vi "Topo & GridSpectr_DriftCorrection_v8.vi"(6 "Internal use":string, 7 "Grid param":T2 {"height (m)" format="%#_6p"; "width (m)" format="%#_6p"; "center Y (m)" format="%#_6p"; "center X (m)" format="%#_6p"}, 8 "Error in (no error)":errorcluster, 9 "Points Y/Index Y":i32, 10 "Points X/Index X":i32, 11 "Method":enum16{"init", "run", "end"}(ring)=enum."end") -> (0 "Error out":errorcluster)   [LabVIEW 2014]
doc: "Example of a measurement VI to be used in the \"Experiments on a Grid\" tool as external VI.\n\nThis example measure the topography and spectroscopy data. The spectroscopy measurements are taken on a subgrid. The data are saved to a sxm and a binary file.\n\n- Nanonis Programming Interface -"
uses:
  <userlib>/Nanonis Prog Interface V5/Nanonis Prog Interface.lvlib
  <userlib>/Nanonis Prog Interface V5/Scan/Grid/GridPatternGet.vi
panel:
  out "Progress":u8(slide) scale=0.0..100.0 scale format="%#.1g"
  out "total Points":i32
  in  "preSTS delay [ms]":u32=3
  in  "STS Bias":dbl=0.005 format="%#_6p"
  in  "Move Bias":dbl=-0.01 format="%#_6p"
  in  "Move Current":dbl=1.5e-11 format="%#_6p"
  in  "Imaging Bias":dbl=-0.01 format="%#_6p"
  in  "max applied Drift Correction":i32=20 min=1 max=100 step=1 format="%.0p"
  in  "Correlate":u16(ring) items=["first Frame", "successive Frames"]
  out "Topo Images taken":i32=14
  in  "Increment":i32=40
  in  "Threshold":i32=2 min=1 step=1
  in  "tip Speed (m/s)":sgl=1e-08 format="%.2p"
  in  "Drift Correction 2":T1
  out "X drift":i32
  out "Y drift":i32
  out "Last Drift detected":i32=40
  in  "MaxImagesBack":i32=40
  in  "Channel index (0-23)":u8=14
  in  "File name":string="single_mol_shortSTS"
  in  "STS Current":dbl=1.15e-09 format="%#_6p"
  in  "Imaging Current":dbl=1.5e-11 format="%#_6p"
  in  "zdrift \nDuration (s)":dbl
  in  "Correct z drift":bool
  out "Status":string="finishing"
  in  "Drift correction Pixels":i32=256 caption="Topo Pixels"
  out "Y Offset":dbl format="%#_6p"
  out "X Offset":dbl format="%#_6p"
  out "Points taken":dbl=14.0
  in  "Drift Correction every":i32=40
  in  "Y subgrid spacing":u16=1
  in  "X subgrid spacing":u16=1
  # "GRID points"
  # "Increase this if no Drift was detected for \na certain number of images"
  # "images back"
  # "% of image size"
  # "RUN smart tilt before starting the GRID"
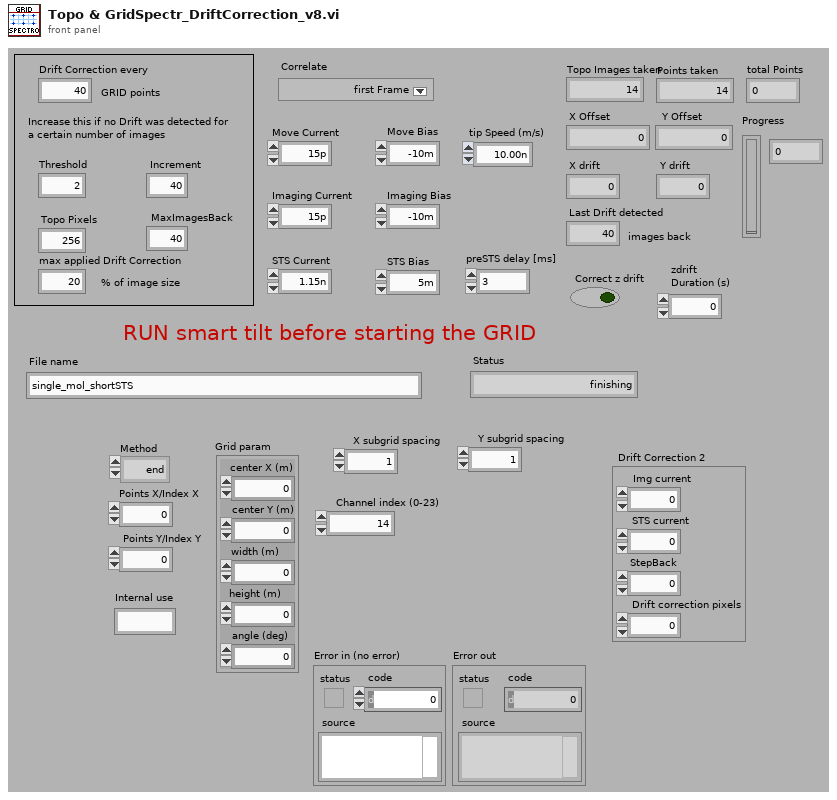
[diagram p1: front panel]
types:
  T1 = cluster{"Img current":dbl, "STS current":dbl, "StepBack":dbl, "Drift correction pixels":dbl}
  T2 = cluster{"center X (m)":sgl, "center Y (m)":sgl, "width (m)":sgl, "height (m)":sgl, "angle (deg)":sgl}
  T3 = cluster{"center X":sgl, "center Y":sgl, "angle":sgl, "width":sgl, "height":sgl, "# pixels":i32, "# lines":i32}
  T4 = cluster{"Name":string, "Calibration":sgl, "Offset":sgl, "Channel index":i32}[]
  T5 = cluster{"up/down":bool, "time/line":sgl, "start time":timestamp, "end time":timestamp}
  T6 = cluster{"Z averaging time (s)":sgl, "Z offset (m)":sgl, "Initial settling time (s)":sgl}
  T7 = cluster{"Max. slew rate (V/s)":sgl, "Settling time (s)":sgl, "Integration time (s)":sgl}
  T8 = cluster{"End settling time (s)":sgl, "Z control time (s)":sgl}
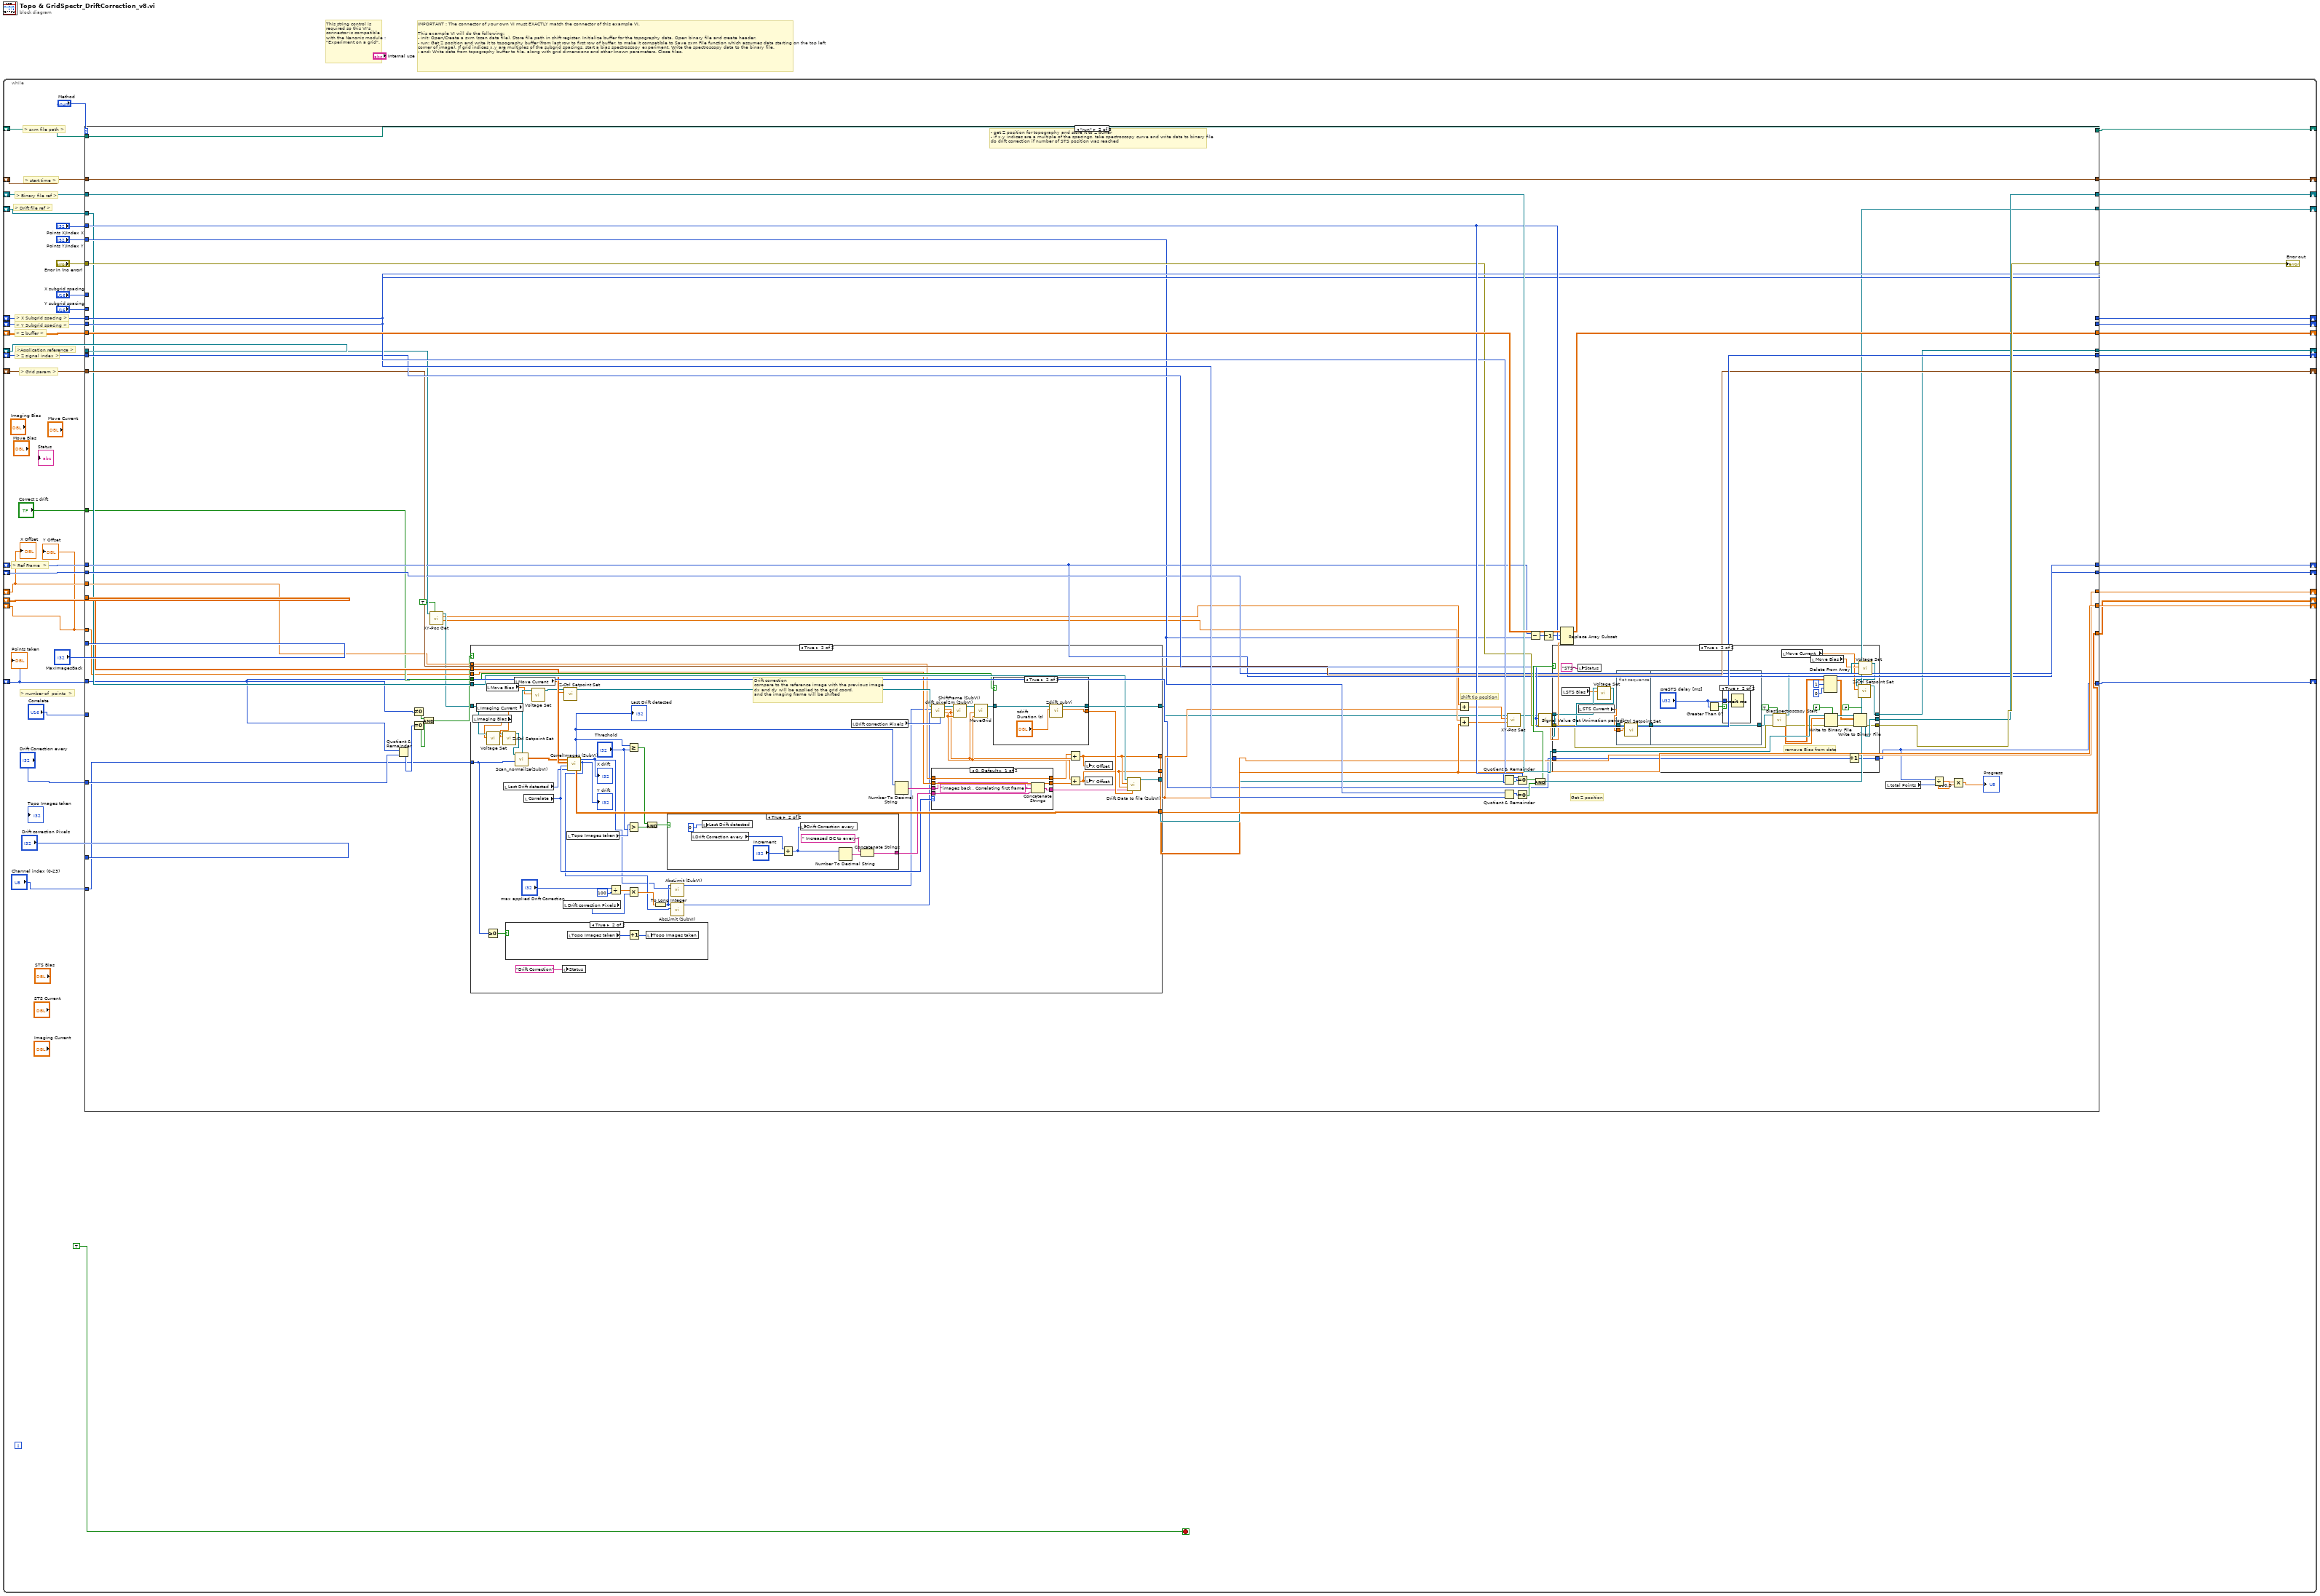
[diagram p0: block diagram]
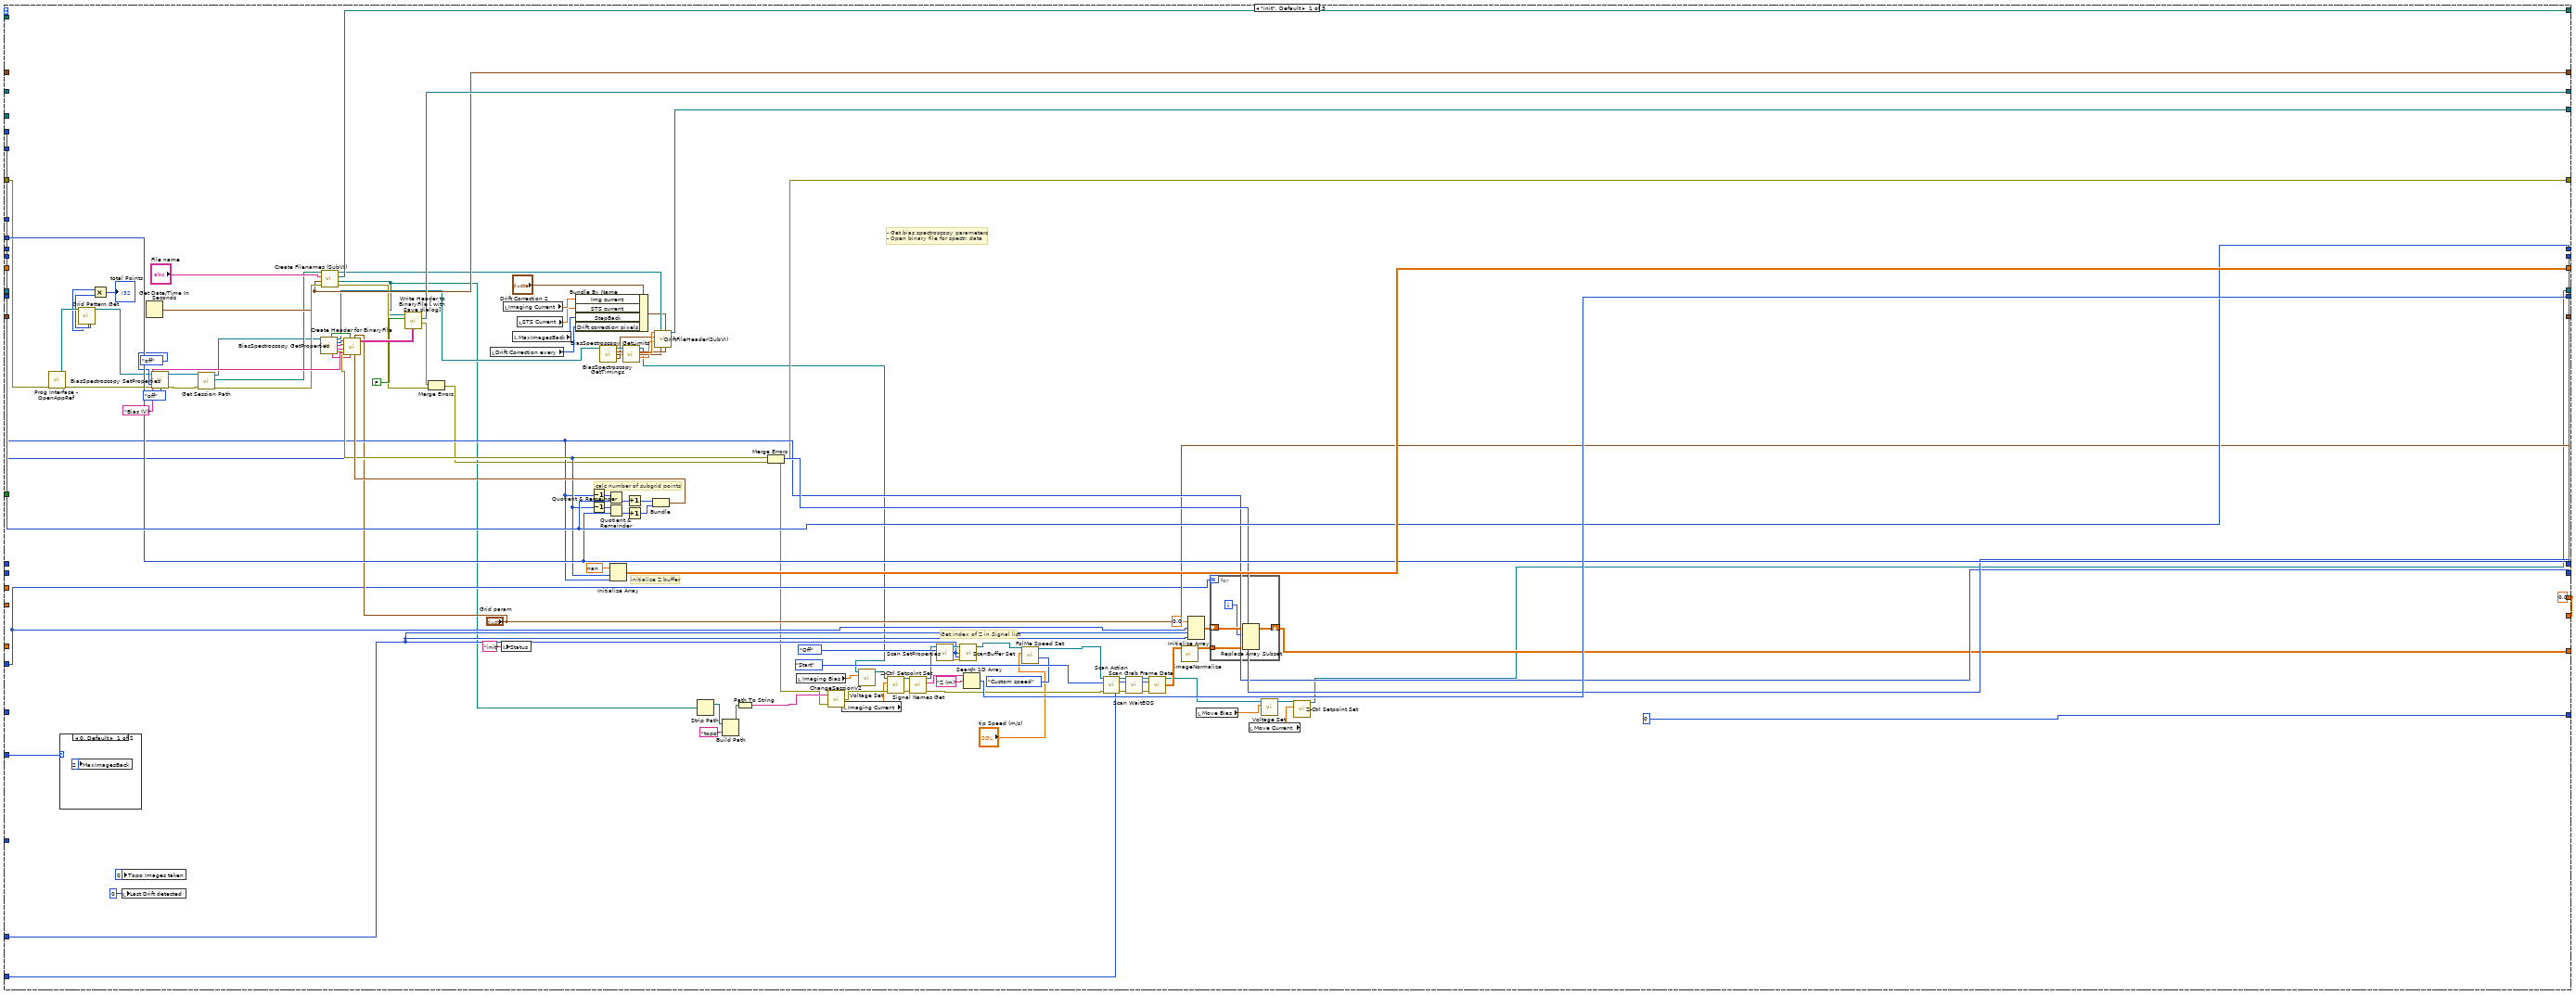
[diagram p2: hidden frame]
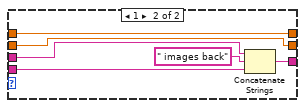
[diagram p5: hidden frame]
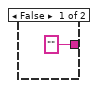
[diagram p7: hidden frame]
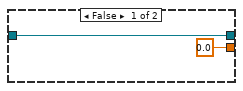
[diagram p8: hidden frame]
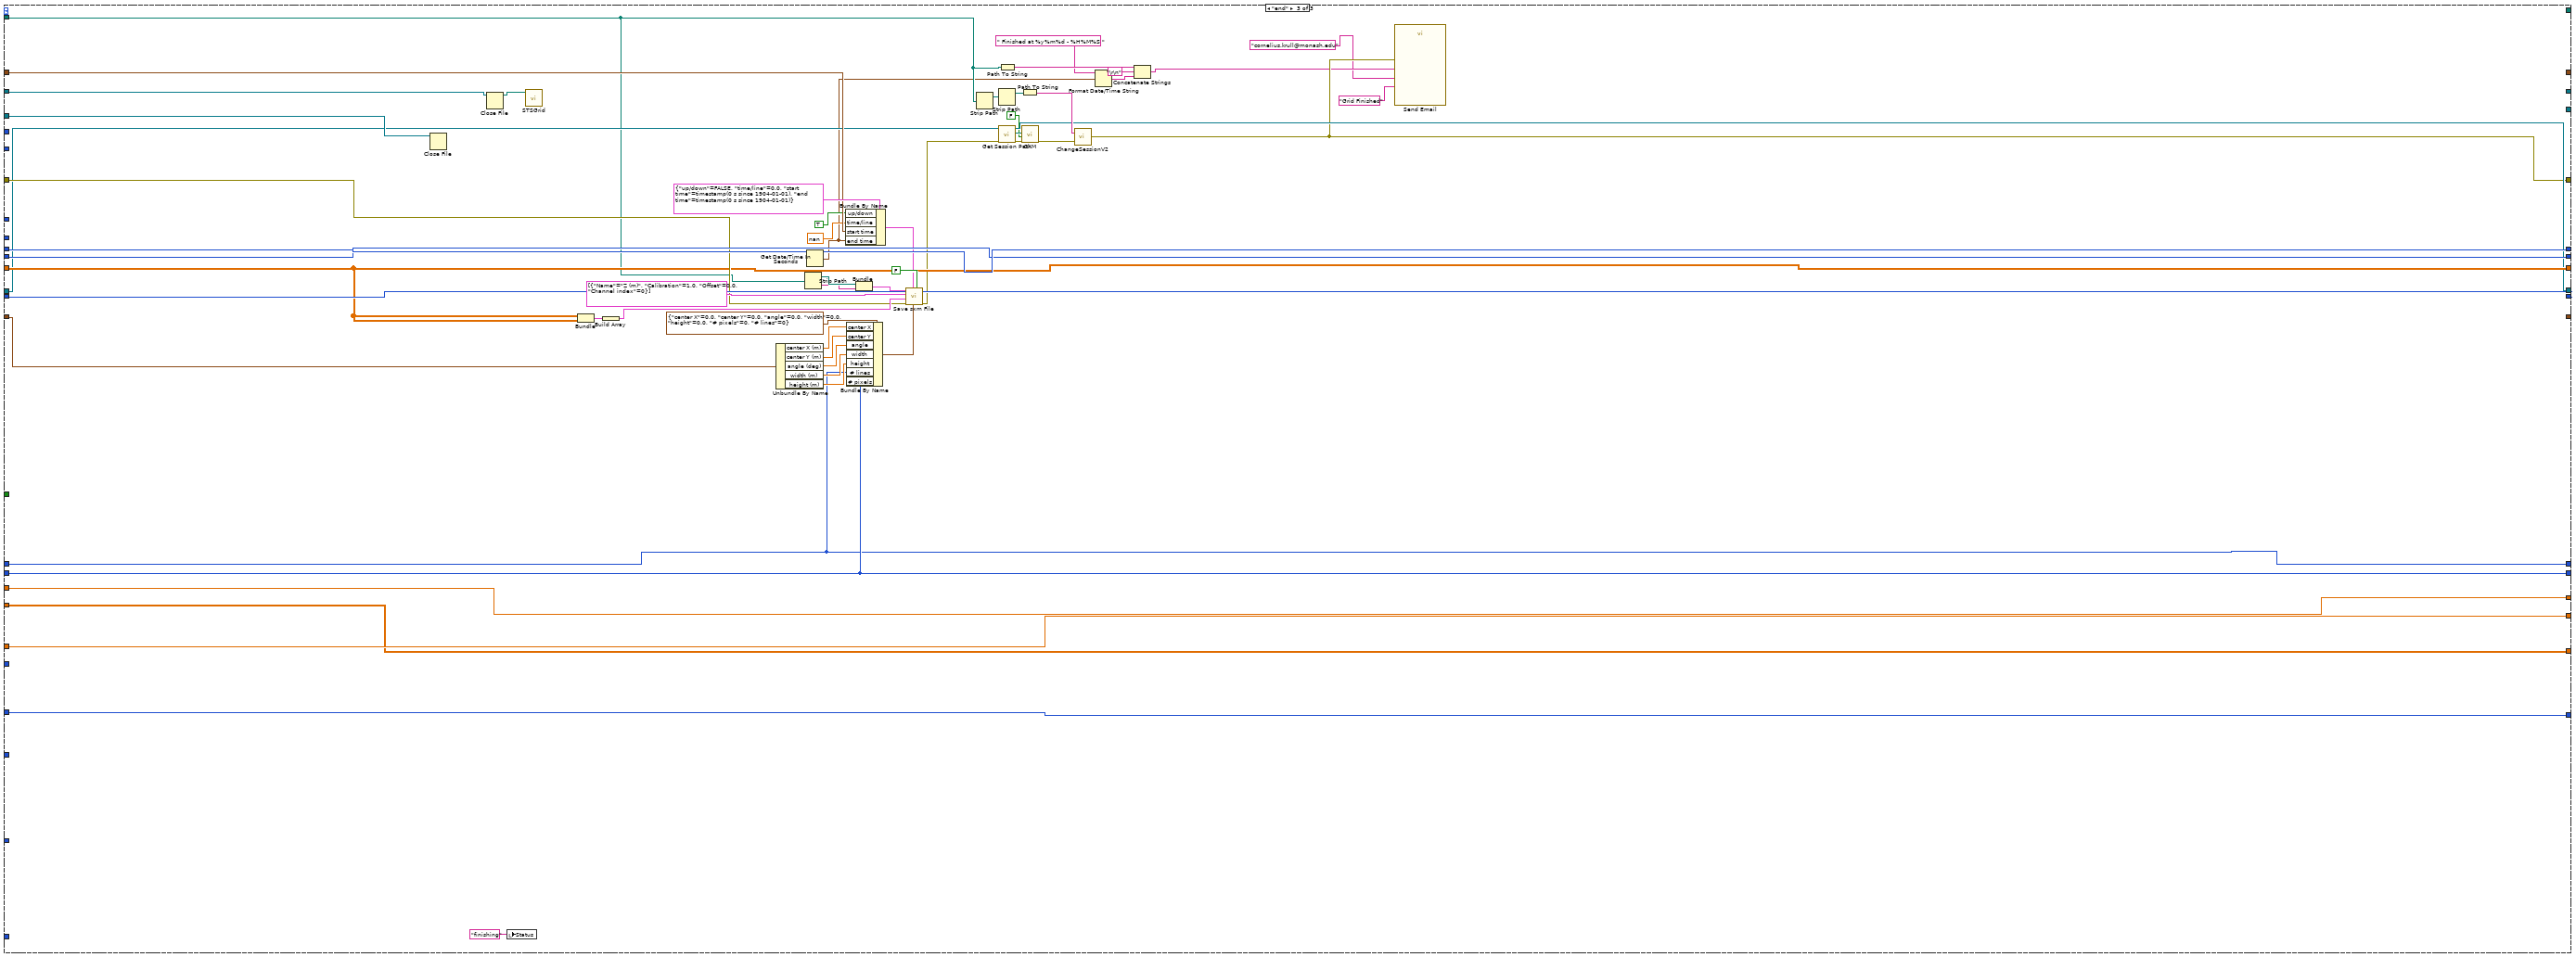
[diagram p11: hidden frame]
diagram:
  # "This string control is required so this VI's connector is compatible with the Nanonis module : \"Experiment on a grid\"."
  # "IMPORTANT : The connector of your own VI must EXACTLY match the connector of this example VI.\n\nThis example VI will do the following:\n- init: Open/Create a sxm (scan data file). Store file path in shift register. Initialize buffer for the topography data. Open binary file and create header.\n- run: Get Z position and write it to topography buffer (from last row to first row of buffer, to make it compatible to Save sxm File function which assumes data starting on the top left corner of image). If grid indices x,y are multiples of the subgrid spacings, start a bias spectroscopy experiment. Write the spectroscopy data to the binary file.\n- end: Write data from topography buffer to file, along with grid dimensions and other known parameters. Close files."
  n1 = while {
    shift-right: [w21] -> _
    shift-left: _ -> [w44]
    shift-right: [w39] -> _
    shift-left: _ -> [w38]
    shift-right: [w36] -> _
    shift-left: _ -> [w37]
    shift-right: [w35] -> _
    shift-left: _ -> [w34]
    shift-right: [w28] -> _
    shift-left: _ -> [w30]
    shift-right: [w29] -> _
    shift-left: _ -> [w31]
    shift-right: [w27] -> _
    shift-left: _ -> [w26]
    shift-right: [w25] -> _
    shift-left: _ -> [w24]
    shift-right: [w23] -> _
    shift-left: _ -> [w22]
    shift-right: [w20] -> _
    shift-left: _ -> [w19]
    shift-right: [w18] -> _
    shift-left: _ -> [w17]
    shift-right: [w16] -> _
    shift-left: _ -> [w9]
    shift-right: [w15] -> _
    shift-left: _ -> [w8]
    shift-right: [w14] -> _
    shift-left: _ -> [w11]
    shift-right: [w13] -> _
    shift-left: _ -> [w10]
    shift-right: [w6] -> _
    shift-left: _ -> [w5]
    stop <- TRUE stop-if-true
    # "> Drift file ref >"
    # "> number of  points  >"
    # "> Ref Frame  >"
    # "> Grid param >"
    # "> start time >"
    # ">Application reference >"
    # "> Y Subgrid spacing >"
    # "> X Subgrid spacing >"
    # "> Z signal index >"
    # "> Binary file ref >"
    # "> Z buffer >"
    # "> sxm file path >"
    n2 = case shown="\"run\"" "Method" {
      tunnel: [w109 w216 _] -> w21
      tunnel: w44 -> [_ w216 w352]
      tunnel: "Error in (no error)" -> [w111 w202 w384]
      tunnel: [w72 w215 w353] -> w42
      tunnel: "Points X/Index X" -> [w130 w210 _]
      tunnel: "Points Y/Index Y" -> [w131 w194 _]
      tunnel: [w154 w213 w373] -> w39
      tunnel: w38 -> [_ w214 w373]
      tunnel: w37 -> [_ w212 w366]
      tunnel: [w146 w211 _] -> w36
      tunnel: [w144 w200 w398] -> w35
      tunnel: w34 -> [_ w200 w398]
      tunnel: "X subgrid spacing" -> [w143 _ _]
      tunnel: "Y subgrid spacing" -> [w142 _ _]
      tunnel: w31 -> [_ w204 w397]
      tunnel: w30 -> [_ w203 w396]
      tunnel: [w143 w204 w397] -> w29
      tunnel: [w142 w203 w396] -> w28
      tunnel: [w60 w187 w358] -> w27
      tunnel: w26 -> [_ w170 w359]
      tunnel: ["Grid param" w197 _] -> w25
      tunnel: w24 -> [_ w197 w383]
      tunnel: [w108 w198 _] -> w23
      tunnel: w22 -> [_ w198 w391]
      tunnel: [w131 w195 w374] -> w20
      tunnel: w19 -> [_ w195 w374]
      tunnel: [w130 w196 w375] -> w18
      tunnel: w17 -> [_ w196 w375]
      tunnel: [w121 w177 w372] -> w16
      tunnel: [w121 w182 w370] -> w15
      tunnel: [w103 w176 w367] -> w14
      tunnel: [0 w164 w371] -> w13
      tunnel: w10 -> [_ w173 w371]
      tunnel: "Drift Correction every" -> [_ w190 _]
      tunnel: w11 -> [_ w181 w367]
      tunnel: w9 -> [_ w188 w372]
      tunnel: w8 -> [_ w174 w370]
      tunnel: "Drift correction Pixels" -> [w102 _ _]
      tunnel: [w98 w179 _] -> w6
      tunnel: w5 -> [_ w180 w368]
      tunnel: "Correct z drift" -> [_ w178 _]
      tunnel: "Channel index (0-23)" -> [w106 w175 _]
      tunnel: "MaxImagesBack" -> [w101 _ _]
      tunnel: "Correlate" -> [w63 _ _]
      frame "init", Default {
        w121 = 0.0
        # "- Get bias spectroscopy parameters\n- Open binary file for spectr. data"
        # "initialize Z buffer"
        # "calc number of subgrid points"
        # "Get index of Z in Signal list"
        n3 = call <userlib>:"Prog Interface - OpenAppRef.vi"("Error in (no error)"=w111) -> ("Error out"=w70:errorcluster, "Application reference"=w51:refnum<vi>)  [unwired: 5 in]
        n4 = case shown="0, Default" w63 {
          frame 0, Default {
            n5 = local write "MaxImagesBack"(2 ("StepsBack")) -> ()
          }
          frame 1 {
          }
        }
        n6 = call-poly <userlib>:"Grid Pattern Get.vi"("Application ref in"=w51) -> ("Points Y"=w48:i32, "Points X"=w49:i32, "Application ref out"=w50:refnum<vi>)  [unwired: 10 in, 6 out]
        n7 = Multiply(x=w48, y=w49) -> (x*y=→"total Points":i32)
        n8 = local write "Topo Images taken"(0 ("Images taken")) -> ()
        n9 = local write "Last Drift detected"(0 ("Last Drift detected")) -> ()
        n10 = Get Date/Time In Seconds() -> (seconds since 1Jan1904=w108:timestamp)
        n11 = call <userlib>:"BiasSpectroscopy SetProperties.vi"("Application ref in"=w50, "Autosave (no change)"=enum16{"no change", "on", "off"}."off", "Error in (no error)"=w70, "Save dialog"=enum16{"no change", "on", "off"}."off") -> ("Application ref out"=w66:refnum<vi>, "Error out"=w65:errorcluster)  [unwired: 10 in]
        n12 = call <userlib>:"Get Session Path.vi"("error in (no error)"=w65, "Application ref in"=w66) -> ("error out"=w110:errorcluster, "Session path"=w78:path, "Application ref out"=w67:refnum<vi>)  [unwired: 7 in]
        n13 = call <userlib>:"BiasSpectroscopy GetProperties.vi"("Application ref in"=w67) -> ("Backward sweep"=w150:bool, "Application ref out"=w82:refnum<vi>, "Number of points"=w133:i32, "Channels"=w132:string[], "Parameters"=w148:string[], "Fixed parameters"=w135:string[], "Error out"=w147:errorcluster)  [unwired: 6 in, 2 out]
        n14 = call "Create Filenames (SubVI).vi"("error in (no error)"=w110, "seconds since 1Jan1904"=w108, "File name"="File name", "Session path"=w78) -> ("error out"=w83:errorcluster, "binFilePath"=w74:path, "topoFilePath"=w109:path, "Drift File out"=w99:refnum<file>)  [unwired: 4 in]
        n15 = local read "Drift Correction every"() -> (w93:i32)
        n16 = local write "Status"("init" ("Status")) -> ()
        n17 = local read "Imaging Current"() -> (w95:dbl)
        n18 = local read "MaxImagesBack"() -> (w92:i32)
        n19 = local read "STS Current"() -> (w94:dbl)
        n20 = Bundle By Name(cluster="Drift Correction 2", "Img current"=w95, "STS current"=w94, "StepBack"=w92, "Drift correction pixels"=w93) -> (w96:T1)
        n21 = Decrement(x=w130) -> (x-1=w141:i32)
        n22 = Decrement(x=w131) -> (x-1=w140:i32)
        n23 = call <userlib>:"BiasSpectroscopy GetTimings.vi"("Application ref in"=w82) -> ("Application ref out"=w91:refnum<vi>, "Initialization"=w88:T6, "Sweep Timing"=w86:T7, "End of Sweep"=w87:T8)  [unwired: 10 in, 1 out]
        n24 = Quotient & Remainder(x=w141, y=w143) -> (floor(x/y)=w139:i32)  [unwired: 1 out]
        n25 = Quotient & Remainder(x=w140, y=w142) -> (floor(x/y)=w138:i32)  [unwired: 1 out]
        n26 = Initialize Array(sgl nan ("element"), w131, w130) -> (w154:sgl[][])
        n27 = call <userlib>:"BiasSpectroscopy GetLimits.vi"("Application ref in"=w91) -> ("End value (V)"=w89:sgl, "Start value (V)"=w90:sgl, "Application ref out"=w58:refnum<vi>)  [unwired: 5 in, 1 out]
        n28 = Increment(x=w139) -> (x+1=w137:i32)
        n29 = Increment(x=w138) -> (x+1=w136:i32)
        n30 = Bundle(w137, w136) -> (w149:cluster{i32, i32})  [unwired: 1 in]
        n31 = call <userlib>:"Create Header for BinaryFile.vi"("Grid points"=w149, "Grid param"="Grid param", "Fixed parameters"=w135, "Backward sweep"=w150, "Sweep signal"="Bias (V)" ("Sweep Signal"), "Parameters"=w148, "Channels"=w132, "Points per sweep"=w133) -> ("Header (fixed attributes)"=w152:string[][])  [unwired: 3 in]
        n32 = call <userlib>:"Write Header to BinaryFile [ with Save dialog].vi"("Fixed Attributes"=w152, "Show Dialog? (T)"=FALSE, "Filename"=w74) -> ("Error out"=w84:errorcluster, "File ref"=w146:refnum<file>)  [unwired: 5 in, 2 out]
        n33 = Merge Errors(w84, w83) -> (w85:errorcluster)
        n34 = call "DriftFileHeader(SubVI).vi"("Initialization"=w88, "Drift Correction"=w96, "Sweep Timing"=w86, "Byte Stream File in"=w99, "End value (V)"=w89, "End of Sweep"=w87, "Start value (V)"=w90) -> ("Byte Stream File out"=w98:refnum<file>)  [unwired: 4 in]
        n35 = Strip Path(path=w74) -> (stripped path=w77:path)  [unwired: 1 out]
        n36 = Build Path(base path=w77, name or relative path="topo") -> (appended path=w75:path)
        n37 = Path To String(path=w75) -> (string=w73:string)
        n38 = Merge Errors(w147, w85) -> (w72:errorcluster)
        n39 = local read "Imaging Bias"() -> (w54:dbl)
        n40 = call "ChangeSessionV2.vi"("error in (no error)"=w72, "Session"=w73) -> ("error out"=w71:errorcluster)
        n41 = local read "Imaging Current"() -> (w53:dbl)
        n42 = call <userlib>:"Voltage Set.vi"("Bias (V)"=w54, "Application ref in"=w58) -> ("Application ref out"=w57:refnum<vi>)  [unwired: 8 in, 1 out]
        n43 = call <userlib>:"Z-Ctrl Setpoint Set.vi"("error in (no error)"=w71, "Z Controller setpoint"=w53, "Application ref in"=w57) -> ("error out"=w112:errorcluster, "Application ref out"=w113:refnum<vi>)  [unwired: 7 in]
        n44 = call <userlib>:"Signal Names Get.vi"("error in (no error)"=w112, "Application ref in"=w113) -> ("error out"=w122:errorcluster, "Signals Names"=w134:string[], "Application ref out"=w117:refnum<vi>)  [unwired: 5 in]
        n45 = call <userlib>:"Scan SetProperties.vi"("Application ref in"=w117, "Continuous scan"=enum16{"No change", "On", "Off"}."Off") -> ("Application ref out"=w119:refnum<vi>, "Error out"=w118:errorcluster)  [unwired: 12 in]
        n46 = call <userlib>:"ScanBuffer Set.vi"("Application ref in"=w119, "Pixels"=w102, "Lines"=w102, "error in (no error)"=w118) -> ("Application ref out"=w61:refnum<vi>)  [unwired: 10 in, 1 out]
        n47 = Search 1D Array(1D array=w134, element="Z (m)") -> (index of element=w144:i32)  [unwired: 1 in]
        n48 = call <userlib>:"FolMe Speed Set.vi"("Speed Setting (Custom)"=enum32{"Scan speed", "Custom speed"}."Custom speed", "Speed (m/s)"="tip Speed (m/s)", "Application ref in"=w61) -> ("Application ref out"=w81:refnum<vi>)  [unwired: 5 in, 1 out]
        n49 = call <userlib>:"Scan Action.vi"("error in (no error)"=w122, "Scan action (Start)"=enum16{"Start", "Stop", "Pause", "Resume"}."Start", "Application ref in"=w81) -> ("error out"=w128:errorcluster, "Application ref out"=w127:refnum<vi>)  [unwired: 6 in]
        n50 = call <userlib>:"Scan WaitEOS.vi"("error in (no error)"=w128, "Application ref in"=w127) -> ("error out"=w125:errorcluster, "Application ref out"=w126:refnum<vi>)  [unwired: 5 in, 2 out]
        n51 = call <userlib>:"Scan Grab Frame Data.vi"("Application ref in"=w126, "Channel index (0-23)"=w106, "error in (no error)"=w125) -> ("Application ref out"=w52:refnum<vi>, "Scan frame data"=w114:sgl[][])  [unwired: 8 in, 3 out]
        n52 = call "imageNormalize.vi"("Data"=w114) -> ("Array"=w100:dbl[][])  [unwired: 10 in]
        n53 = Initialize Array(0.0 ("element"), w101, w102, w102) -> (w104:dbl[][][])
        n54 = local read "Move Bias"() -> (w56:dbl)
        n55 = for {
          N: w101 -> [_]
          tunnel: w100 -> [w158]
          shift-right: [w157] -> w103
          shift-left: w104 -> [w159]
          i -> [w156]
          n56 = Replace Array Subset(array=w159, new element=w158, index (dim 0)=w156) -> (w157:dbl[][][])  [unwired: 2 in]
        }
        n57 = local read "Move Current"() -> (w55:dbl)
        n58 = call <userlib>:"Voltage Set.vi"("Bias (V)"=w56, "Application ref in"=w52) -> ("Application ref out"=w59:refnum<vi>)  [unwired: 8 in, 1 out]
        n59 = call <userlib>:"Z-Ctrl Setpoint Set.vi"("Z Controller setpoint"=w55, "Application ref in"=w59) -> ("Application ref out"=w60:refnum<vi>)  [unwired: 8 in, 1 out]
      }
      frame "run" {
        # "shift tip position"
        # "Get Z position"
        # "- get Z position for topography and store it to Z buffer\n- if x,y indices are a multiple of the spacings, take spectroscopy curve and write data to binary file\ndo drift correction if number of STS position was reached"
        n60 = Quotient & Remainder(x=w173, y=w190) -> (x-y*floor(x/y)=w191:i32)  [unwired: 1 out]
        n61 = Not Equal To 0?(x=w173) -> (x != 0?=w171:bool)
        n62 = Equal To 0?(x=w191) -> (x = 0?=w189:bool)
        n63 = And(x=w171, y=w189) -> (x .and. y?=w172:bool)
        n64 = call <userlib>:"XY-Pos Get.vi"("Wait for newest data (F=False)"=TRUE, "Application ref in"=w170) -> ("Y (m)"=w166:sgl, "X (m)"=w167:sgl, "Application ref out"=w169:refnum<vi>)  [unwired: 5 in, 1 out]
        n65 = case shown="True" w172 {
          tunnel: w169 -> [w221 w229]
          tunnel: [w221 w271] -> w165
          tunnel: w181 -> [w218 w266]
          tunnel: [w220 w269] -> w177
          tunnel: [w219 w268] -> w182
          tunnel: w188 -> [w220 w245]
          tunnel: w174 -> [w219 w243]
          tunnel: [w218 w262] -> w176
          tunnel: w180 -> [w217 w274]
          tunnel: [w217 w273] -> w179
          tunnel: w178 -> [_ w270]
          tunnel: w175 -> [_ w249]
          frame False {
          }
          frame True {
            # "Drift correction \ncompare to the reference image with the previous image \ndx and dy will be applied to the grid coord, \nand the imaging frame will be shifted"
            n66 = local read "Imaging Bias"() -> (w227:dbl)
            n67 = local read "Imaging Current"() -> (w226:dbl)
            n68 = local read "Move Bias"() -> (w223:dbl)
            n69 = Greater Or Equal To 0?(x=w249) -> (x >= 0?=w248:bool)
            n70 = call <userlib>:"Voltage Set.vi"("Bias (V)"=w227, "Application ref in"=w229) -> ("Application ref out"=w228:refnum<vi>)  [unwired: 8 in, 1 out]
            n71 = call <userlib>:"Z-Ctrl Setpoint Set.vi"("Z Controller setpoint"=w226, "Application ref in"=w228) -> ("Application ref out"=w267:refnum<vi>)  [unwired: 8 in, 1 out]
            n72 = local read "Last Drift detected"() -> (w240:i32)
            n73 = case shown="True" w248 {
              frame False {
              }
              frame True {
                n74 = local read "Topo Images taken"() -> (w289:i32)
                n75 = Increment(x=w289) -> (x+1=w288:i32)
                n76 = local write "Topo Images taken"(w288) -> ()
              }
            }
            n77 = local read "Move Current"() -> (w222:dbl)
            n78 = call "Scan_normailze(SubVI).vi"("Channel index (0-23)"=w249, "Application in"=w267) -> ("Array"=w263:dbl[][], "Application out"=w224:refnum<vi>)  [unwired: 7 in, 1 out]
            n79 = local read "Correlate"() -> (w246:u16)
            n80 = call <userlib>:"Voltage Set.vi"("Bias (V)"=w223, "Application ref in"=w224) -> ("Application ref out"=w225:refnum<vi>)  [unwired: 8 in, 1 out]
            n81 = local write "Status"("Drift Correction" ("Status")) -> ()
            n82 = local read "Drift correction Pixels"() -> (w237:i32)
            n83 = call <userlib>:"Z-Ctrl Setpoint Set.vi"("Z Controller setpoint"=w222, "Application ref in"=w225) -> ("Application ref out"=w258:refnum<vi>)  [unwired: 8 in, 1 out]
            n84 = local read "Topo Images taken"() -> (w251:i32)
            n85 = call "CorrelImages (SubVI).vi"("last drift detected"=w240, "Correlate"=w246, "Ref Array"=w266, "New Image"=w263) -> ("Y drift"=w234:i32, "X drift"=w231:i32, "Ref Array out"=w262:dbl[][][], "Queue Steps"=w247:i32)  [unwired: 4 in]
            "X drift" <- w231
            "Y drift" <- w234
            "Last Drift detected" <- w247
            n86 = Divide(x="max applied Drift Correction", y=100) -> (x/y=w236:dbl)
            n87 = Greater Or Equal?(x=w247, y="Threshold") -> (x >= y?=w253:bool)
            n88 = Greater?(x=w251, y="Threshold") -> (0:w250:bool)
            n89 = Multiply(x=w236, y=w237) -> (x*y=w238:dbl)
            n90 = And(x=w253, y=w250) -> (x .and. y?=w252:bool)
            n91 = To Long Integer(number=w238) -> (32bit integer=w230:i32)
            n92 = case shown="True" w252 {
              tunnel: ["" w293] -> w254
              frame False {
              }
              frame True {
                n93 = local read "Drift Correction every"() -> (w292:i32)
                n94 = local write "Last Drift detected"(0 ("Last Drift detected")) -> ()
                n95 = Add(x=w292, y="Increment") -> (x+y=w296:i32)
                n96 = local write "Drift Correction every"(w296) -> ()
                n97 = Number To Decimal String(number=w296) -> (decimal integer string=w295:string)  [unwired: 1 in]
                n98 = Concatenate Strings(" Increased DC to every " ("string"), w295) -> (w293:string)
              }
            }
            n99 = call "AbsLimit (SubVI).vi"("in"=w231, "Abslimt"=w230) -> ("Numeric out"=w233:i32)  [unwired: 9 in]
            n100 = call "AbsLimit (SubVI).vi"("in"=w234, "Abslimt"=w230) -> ("Numeric out"=w232:i32)  [unwired: 9 in]
            n101 = local read "Drift correction Pixels"() -> (w259:i32)
            n102 = Number To Decimal String(number=w247) -> (decimal integer string=w265:string)  [unwired: 1 in]
            n103 = call "drift_pixel2m (SubVI).vi"("Application in"=w258, "X drift"=w233, "Y drift"=w232, "Drift correction Pixels"=w259) -> ("Application out"=w257:refnum<vi>, "x drift"=w255:sgl, "y drift"=w256:sgl)  [unwired: 2 in, 1 out]
            n104 = case shown="0, Default" w246 {
              tunnel: w265 -> [w276 w287]
              tunnel: [w281 w286] -> w264
              tunnel: w254 -> [w279 w284]
              tunnel: w245 -> [w277 w283]
              tunnel: [w277 w283] -> w244
              tunnel: w243 -> [w278 w282]
              tunnel: [w278 w282] -> w242
              frame 0, Default {
                n105 = Concatenate Strings(w276, "images back , Correlating first frame " ("string"), w279) -> (w281:string)
              }
              frame 1 {
                n106 = Concatenate Strings(w287, " images back" ("string"), w284) -> (w286:string)
              }
            }
            n107 = call "ShiftFrame (SubVI).vi"("Y shift"=w256, "X shift"=w255, "Application in"=w257) -> ("Application out"=w261:refnum<vi>)  [unwired: 8 in]
            n108 = call "MoveGrid.vi"("y"=w256, "x"=w255, "Application ref in"=w261) -> ("Application ref out"=w260:refnum<vi>)  [unwired: 7 in, 1 out]
            n109 = case shown="True" w270 {
              tunnel: [0.0 ("z drift") w303] -> w272
              tunnel: w260 -> [w298 w302]
              tunnel: [w298 w301] -> w271
              frame False {
              }
              frame True {
                n110 = call "Zdrift_subVi.vi"("Duration"="zdrift \nDuration (s)", "Application in"=w302) -> ("z drift"=w303:dbl, "Application out"=w301:refnum<vi>)  [unwired: 7 in, 1 out]
              }
            }
            n111 = Add(x=w244, y=w255) -> (x+y=w269:dbl)
            n112 = Add(x=w256, y=w242) -> (x+y=w268:dbl)
            n113 = local write "X Offset"(w269) -> ()
            n114 = local write "Y Offset"(w268) -> ()
            n115 = call "Drift Data to file (SubVI).vi"("z drift"=w272, "Comment"=w264, "y Drift"=w268, "X drift"=w269, "Byte Stream File in"=w274) -> ("Byte Stream File out"=w273:refnum<file>)  [unwired: 6 in]
          }
        }
        n116 = Add(x=w167, y=w177) -> (x+y=w184:dbl)
        n117 = Add(x=w166, y=w182) -> (x+y=w183:dbl)
        n118 = Quotient & Remainder(x=w210, y=w204) -> (x-y*floor(x/y)=w209:i32)  [unwired: 1 out]
        n119 = Quotient & Remainder(x=w194, y=w203) -> (x-y*floor(x/y)=w208:i32)  [unwired: 1 out]
        n120 = call <userlib>:"XY-Pos Set.vi"("Y (m)"=w183, "X (m)"=w184, "Application ref in"=w165) -> ("Application ref out"=w185:refnum<vi>)  [unwired: 5 in, 1 out]
        n121 = Equal To 0?(x=w209) -> (x = 0?=w207:bool)
        n122 = Equal To 0?(x=w208) -> (x = 0?=w206:bool)
        n123 = Subtract(x=w195, y=w194) -> (x-y=w193:i32)
        n124 = And(x=w207, y=w206) -> (x .and. y?=w205:bool)
        n125 = call <userlib>:"Signal Value Get (Animation period).vi"("error in (no error)"=w202, "Signal index (0-47)"=w200, "Application ref in"=w185) -> ("error out"=w201:errorcluster, "Signal value"=w199:sgl, "Application ref out"=w186:refnum<vi>)  [unwired: 5 in]
        n126 = Decrement(x=w193) -> (x-1=w192:i32)
        n127 = case shown="True" w205 {
          tunnel: [w306 w322] -> w215
          tunnel: w212 -> [w307 w336]
          tunnel: [w307 w334] -> w211
          tunnel: w201 -> [w306 w333]
          tunnel: w186 -> [w305 w318]
          tunnel: [w305 w310] -> w187
          tunnel: [w304 w320] -> w164
          tunnel: w173 -> [w304 w321]
          frame False {
            # "Point indices aren't multiple of subgrid spacing\n=> no spectroscopy at this point"
          }
          frame True {
            # "remove Bias from data"
            n128 = local read "STS Bias"() -> (w315:dbl)
            n129 = local write "Status"("STS" ("Status")) -> ()
            n130 = local read "STS Current"() -> (w314:dbl)
            n131 = call <userlib>:"Voltage Set.vi"("Bias (V)"=w315, "Application ref in"=w318) -> ("Application ref out"=w317:refnum<vi>)  [unwired: 8 in, 1 out]
            n132 = flat-sequence {
              tunnel: w317 -> [w339]
              tunnel: w314 -> [w337]
              tunnel: [w338] -> w313
              tunnel: [w342] -> w316
              tunnel: w313 -> [w342]
              frame #0 {
                n133 = call <userlib>:"Z-Ctrl Setpoint Set.vi"("Z Controller setpoint"=w337, "Application ref in"=w339) -> ("Application ref out"=w338:refnum<vi>)  [unwired: 8 in, 1 out]
              }
              frame #1 {
                n134 = Greater Than 0?(x="preSTS delay [ms]") -> (x > 0?=w340:bool)
                n135 = case shown="True" w340 {
                  tunnel: "preSTS delay [ms]" -> [_ w343]
                  frame False {
                  }
                  frame True {
                    n136 = Wait (ms)(milliseconds to wait=w343) -> ()  [unwired: 1 out]
                  }
                }
              }
            }
            n137 = call <userlib>:"BiasSpectroscopy Start.vi"("Application ref in"=w316, "Get data (F)"=TRUE ("Get Data (F)"), "Error in (no error)"=w333) -> ("Application ref out"=w312:refnum<vi>, "Data"=w332:sgl[][], "Parameters"=w331:sgl[], "Error out"=w324:errorcluster)  [unwired: 8 in, 1 out]
            n138 = local read "Move Current"() -> (w308:dbl)
            n139 = local read "Move Bias"() -> (w309:dbl)
            n140 = Delete From Array(array=w332, length=1, index (row)=0 ("index")) -> (array with subset deleted=w330:sgl[][])  [unwired: 1 in, 1 out]
            n141 = Write to Binary File(file (use dialog)=w336, data=w331, error in=w324, 5:FALSE ("prepend array or string size? (T)")) -> (refnum out=w335:refnum<file>, error out=w323:errorcluster)  [unwired: 2 in, 1 out]
            n142 = Increment(x=w321) -> (x+1=w320:i32)
            n143 = Write to Binary File(file (use dialog)=w335, data=w330, error in=w323, 5:FALSE ("prepend array or string size? (T)")) -> (refnum out=w334:refnum<file>, error out=w322:errorcluster)  [unwired: 2 in, 1 out]
            n144 = call <userlib>:"Voltage Set.vi"("Bias (V)"=w309, "Application ref in"=w312) -> ("Application ref out"=w311:refnum<vi>)  [unwired: 8 in, 1 out]
            n145 = call <userlib>:"Z-Ctrl Setpoint Set.vi"("Z Controller setpoint"=w308, "Application ref in"=w311) -> ("Application ref out"=w310:refnum<vi>)  [unwired: 8 in, 1 out]
          }
        }
        n146 = Replace Array Subset(array=w214, new element=w199, index (row)=w192, index (col)=w210) -> (w213:sgl[][])
        n147 = local read "total Points"() -> (w163:i32)
        n148 = Divide(x=w164, y=w163) -> (x/y=w162:dbl)
        n149 = Multiply(x=w162, y=100.0) -> (x*y=→"Progress":dbl)
      }
      frame "end" {
        n150 = Close File(refnum=w368) -> ()  [unwired: 1 in, 2 out]
        n151 = Close File(refnum=w366) -> (path=w365:path)  [unwired: 1 in, 1 out]
        n152 = local write "Status"("finishing" ("Status")) -> ()
        n153 = call "STSGrid.vi"("Binary Spectroscopy File"=w365) -> ()  [unwired: 11 in]
        n154 = Bundle(w373, w373) -> (w395:cluster{sgl[][], sgl[][]})  [unwired: 1 in]
        n155 = Build Array(w395) -> (w394:cluster{sgl[][], sgl[][]}[])
        n156 = Unbundle By Name(w383) -> ("center X (m)"=w381:sgl, "center Y (m)"=w380:sgl, "angle (deg)"=w379:sgl, "width (m)"=w378:sgl, "height (m)"=w377:sgl)
        n157 = Strip Path(path=w352) -> (stripped path=w387:path, name=w386:string)
        n158 = Get Date/Time In Seconds() -> (seconds since 1Jan1904=w347:timestamp)
        n159 = Bundle By Name(cluster=T5 {"up/down"=FALSE, "time/line"=0.0, "start time"=timestamp(0 s since 1904-01-01), "end time"=timestamp(0 s since 1904-01-01)} ("Scan param"), "up/down"=TRUE, "time/line"=sgl nan ("input 7"), "start time"=w391, "end time"=w347) -> (w390:T5)
        n160 = Bundle By Name(cluster=T3 {"center X"=0.0, "center Y"=0.0, "angle"=0.0, "width"=0.0, "height"=0.0, "# pixels"=0, "# lines"=0} ("Scanfield"), "center X"=w381, "center Y"=w380, "angle"=w379, "width"=w378, "height"=w377, "# lines"=w374, "# pixels"=w375) -> (w376:T3)
        n161 = Bundle("stripped path"=w387, "name"=w386) -> (w385:cluster{"stripped path":path, "name":string})  [unwired: 1 in]
        n162 = call <userlib>:"Save sxm File.vi"("Auto file naming? (T)"=FALSE, "Scanfield"=w376, "Scan param"=w390, "error in (no error)"=w384, "Channels data"=w394, "Channels config"=T4 [{"Name"="Z (m)", "Calibration"=1.0, "Offset"=0.0, "Channel index"=0}], "Filename control"=w385) -> ("error out"=w360:errorcluster)  [unwired: 2 in, 2 out]
        n163 = Strip Path(path=w352) -> (stripped path=w364:path)  [unwired: 1 out]
        n164 = Strip Path(path=w364) -> (stripped path=w363:path)  [unwired: 1 out]
        n165 = call <userlib>:"Get Session Path.vi"("error in (no error)"=w360, "Application ref in"=w359) -> ("error out"=w355:errorcluster, "Session path"=w357:path, "Application ref out"=w358:refnum<vi>)  [unwired: 7 in]
        n166 = Path To String(path=w352) -> (string=w351:string)
        n167 = Path To String(path=w363) -> (string=w361:string)
        n168 = call "SXM.vi"("Path"=w357, "Delete"=FALSE, "error in"=w355) -> ("error out"=w354:errorcluster)  [unwired: 7 in]
        n169 = call "ChangeSessionV2.vi"("error in (no error)"=w354, "Session"=w361) -> ("error out"=w353:errorcluster)
        n170 = Format Date/Time String(time format string (%c)=" Finished at %y%m%d - %H%M%S ", seconds (now)=w347) -> (date/time string=w346:string)  [unwired: 1 in]
        n171 = Concatenate Strings(w351, "\r\n", w346) -> (w349:string)
        n172 = call "Send Email"("error in"=w353, "Message"=w349, "Subject"="Grid Finished", "Recipients"="cornelius.krull@monash.edu") -> ()  [unwired: 7 in, 1 out]
      }
    }
    "Error out" <- w42
    "Points taken" <- w10
    "X Offset" <- w9
    "Y Offset" <- w8
  }
